vi "Test_eeprom.vi"() -> ()   [LabVIEW 2019]
panel:
  out "Value response 3":u32
  out "Key response 3":u32
  out "Value response 2":u32
  out "Key response 2":u32
  out "Value response":u32
  out "Key response":u32
  in  "Value to be write":u32
  in  "eeprom address":u32
  in  "Address":u8
  in  "COM Port for serial\nconnection. Check device\nmanager.":string
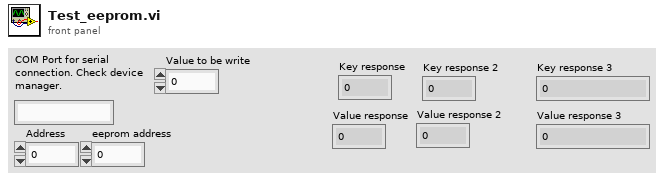
[diagram p1: front panel]
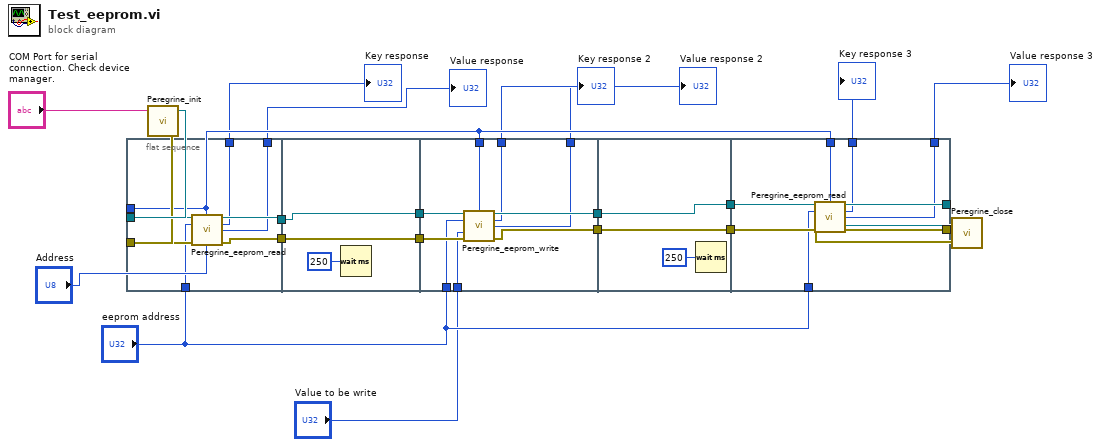
[diagram p0: block diagram]
diagram:
  n1 = flat-sequence {
    tunnel: w21 -> [w30]
    tunnel: [w29] -> w20
    tunnel: w16 -> [w28]
    tunnel: [w27] -> w14
    tunnel: "Address" -> [w26]
    tunnel: "eeprom address" -> [w25]
    tunnel: [w24] -> w6
    tunnel: [w23] -> w5
    tunnel: w20 -> [w33]
    tunnel: [w33] -> w19
    tunnel: [w32] -> w15
    tunnel: w14 -> [w32]
    tunnel: w19 -> [w42]
    tunnel: [w41] -> w18
    tunnel: w15 -> [w40]
    tunnel: [w39] -> w12
    tunnel: "eeprom address" -> [w38]
    tunnel: "Value to be write" -> [w37]
    tunnel: "Address" -> [w36]
    tunnel: [w35] -> w4
    tunnel: [w34] -> w3
    tunnel: w18 -> [w45]
    tunnel: [w45] -> w17
    tunnel: [w44] -> w13
    tunnel: w12 -> [w44]
    tunnel: w17 -> [w53]
    tunnel: w13 -> [w52]
    tunnel: [w51] -> w11
    tunnel: [w50] -> w10
    tunnel: "eeprom address" -> [w49]
    tunnel: "Address" -> [w48]
    tunnel: [w47] -> w2
    tunnel: [w46] -> w1
    frame #0 {
      n2 = call "Peregrine_eeprom_read.vi"("Handle in"=w30, "Address"=w26, "eeprom address"=w25, "error"=w28) -> ("Handle out"=w29:refnum<visa-resource-name>, "Key response"=w24:u32, "Value response"=w23:u32, "error out"=w27:errorcluster)  [unwired: 7 in, 1 out]
    }
    frame #1 {
      n3 = Wait (ms)(milliseconds to wait=u32 250) -> ()  [unwired: 1 out]
    }
    frame #2 {
      n4 = call "Peregrine_eeprom_write.vi"("Handle in"=w42, "Address"=w36, "eeprom address"=w38, "Value to be write"=w37, "error"=w40) -> ("Handle out"=w41:refnum<visa-resource-name>, "Key response"=w35:u32, "Value response"=w34:u32, "error out"=w39:errorcluster)  [unwired: 7 in]
    }
    frame #3 {
      n5 = Wait (ms)(milliseconds to wait=u32 250) -> ()  [unwired: 1 out]
    }
    frame #4 {
      n6 = call "Peregrine_eeprom_read.vi"("Handle in"=w53, "Address"=w48, "eeprom address"=w49, "error"=w52) -> ("Handle out"=w51:refnum<visa-resource-name>, "Key response"=w47:u32, "Value response"=w46:u32, "error out"=w50:errorcluster)  [unwired: 7 in, 1 out]
    }
  }
  n7 = call "Peregrine_init.vi"("COM Port for serial\nconnection. Check device\nmanager."="COM Port for serial\nconnection. Check device\nmanager.") -> ("error out"=w16:errorcluster, "Handle out"=w21:refnum<visa-resource-name>)  [unwired: 3 in]
  n8 = call "Peregrine_close.vi"("error in (no error)"=w10, "Handle in"=w11) -> ()  [unwired: 1 in, 1 out]
  "Key response" <- w6
  "Value response" <- w5
  "Key response 2" <- w4
  "Value response 2" <- w3
  "Key response 3" <- w2
  "Value response 3" <- w1
